vi "Compute Delta Float.vi"(11 "value":dbl) -> (3 "delta":dbl)   [LabVIEW 2014]
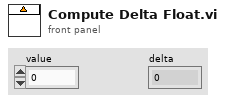
[diagram p1: front panel]
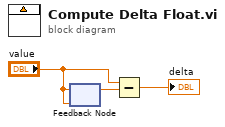
[diagram p0: block diagram]
diagram:
  n1 = feedback #1("value") -> (w1:dbl)
  n2 = feedback-in #1("value") -> ()
  n3 = Subtract(x="value", y=w1) -> (x-y=→"delta":dbl)
